vi "Actor Core.vi"(8 "error in":errorcluster, 11 "Orphan Detector in":refnum<class "Orphan Detector.lvclass">) -> (0 "error out":errorcluster, 3 "Actor out":refnum<class "Actor.lvclass">)   [LabVIEW 2017, in "MGI-Monitored Actor.lvlib" / "Orphan Detector.lvclass"]
doc: "(<B>Filename</B>: Actor Framework.lvlib:Actor.lvclass:Actor Core.vi)\n\nReceives messages to the actor, reacts to them, and initiates any error handling that may shut the actor down.\n\nDescendant classes may override this VI to append parallel tasks for the actor to complete while it handles messages. Overrides use the Call Parent Method node."
uses:
  Orphan Detector.lvclass
  <vilib>/ActorFramework/Actor/Actor.lvclass
  monitored-actor-core/Source/Monitor Data/Actor Data.ctl
  <vilib>/ActorFramework/Message Enqueuer/Message Enqueuer.lvclass
  Orphan Detector.lvclass/Orphan Detector.ctl
  <vilib>/Utility/miscctls.llb/LVRowAndColumnTypeDef.ctl
  <vilib>/ActorFramework/Message/Message.lvclass
  <vilib>/ActorFramework/Message Enqueuer/Message Enqueuer.lvclass/Message Enqueuer.ctl
  <vilib>/ActorFramework/Message Priority Queue/Priority Enqueue.vi
  monitored-actor-core/Source/Monitor Data/Monitor Data.lvclass
panel:
  in  "Poll Rate":i32=500 caption="ms"
  in  "Orphans":i32(listbox)
  # "Orphans"
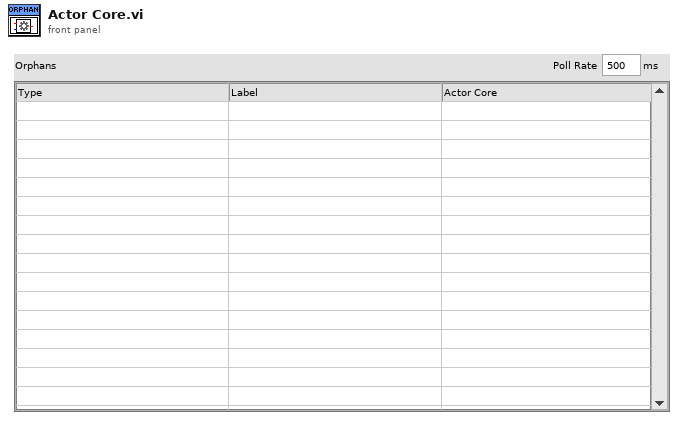
[diagram p1: front panel]
types:
  T1 = enum32{"Invalid", "Standard", "Closed", "Hidden", "Minimized", "Maximized"}
  T2 = typedef "MGI-Monitored Actor Core.lvlib/Monitor Data.lvclass/Actor Data.ctl" = cluster{"Actor Type":string, "Actor Cores":string[], "Self":refnum<class "Message Enqueuer.lvclass">, "Caller":refnum<class "Message Enqueuer.lvclass">, "Actor Label":string, "Last Ping":dbl}
  T3 = typedef "LVRowAndColumnTypeDef.ctl" = cluster{"Row":i32, "Column":i32}
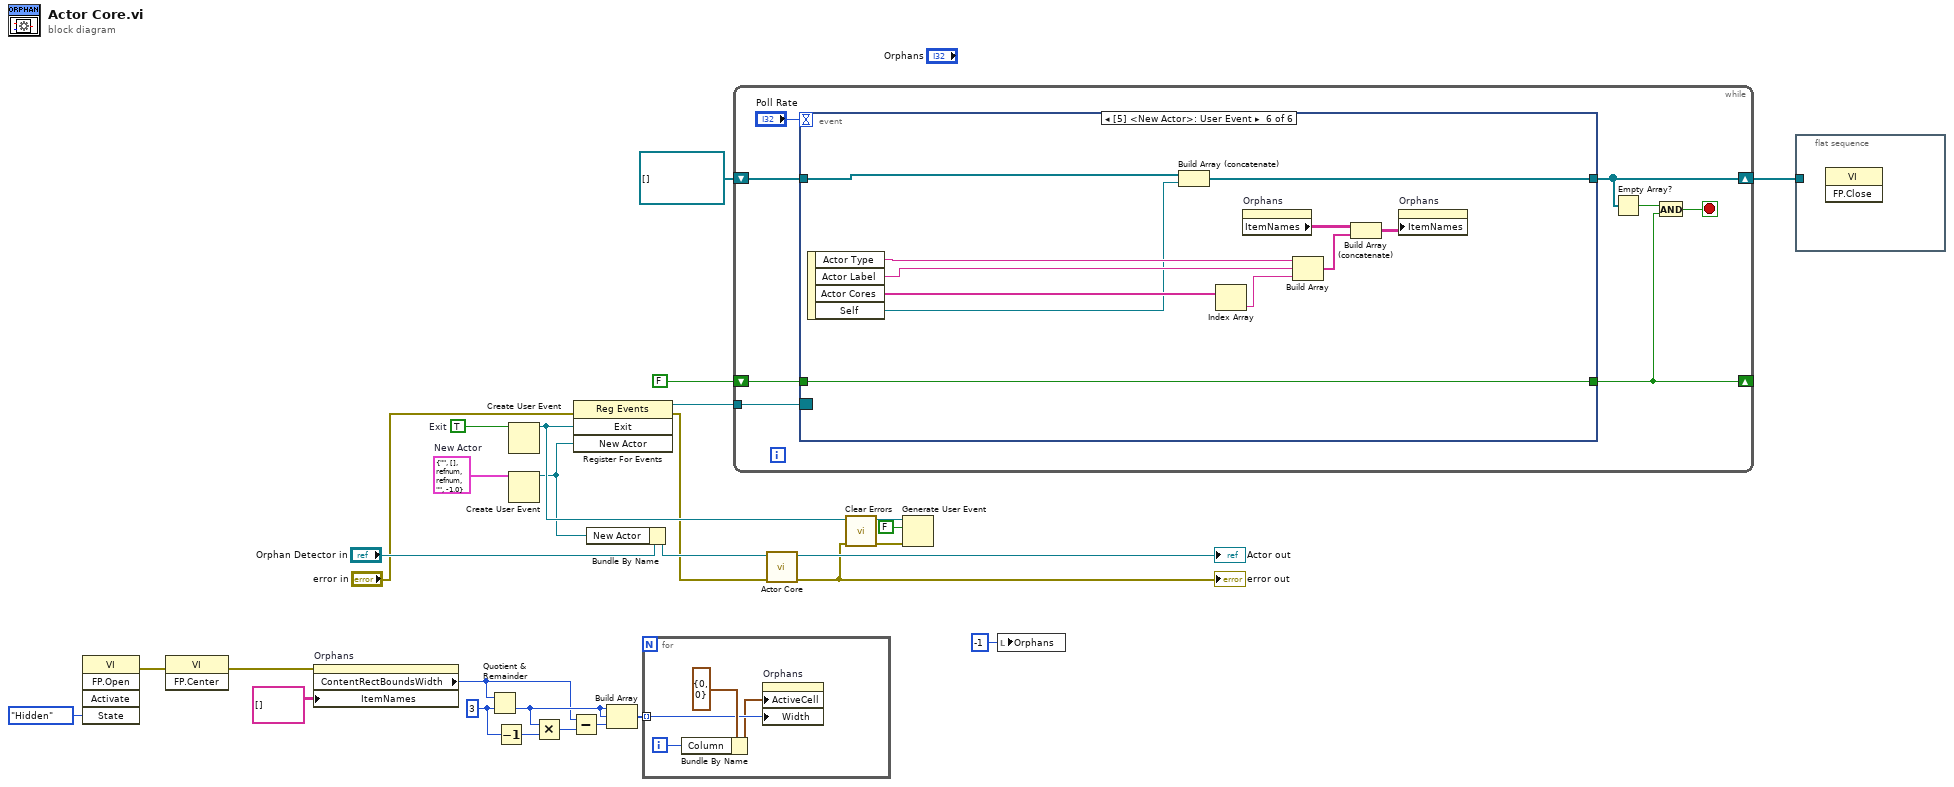
[diagram p0: block diagram]
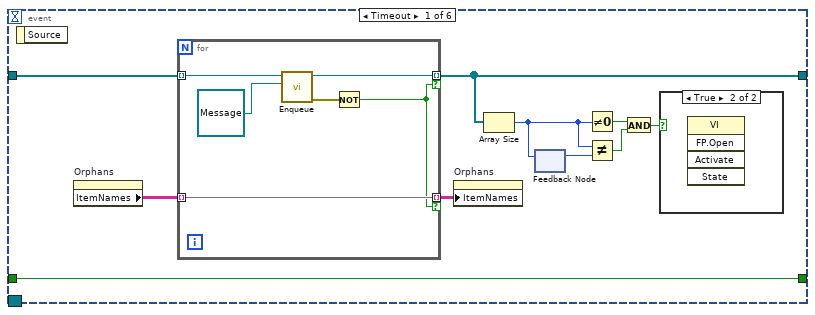
[diagram p2: hidden frame]
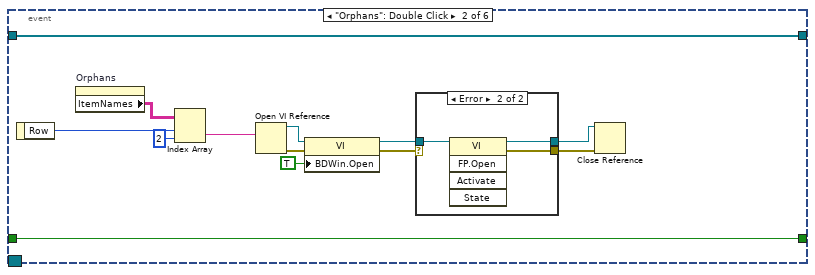
[diagram p4: hidden frame]
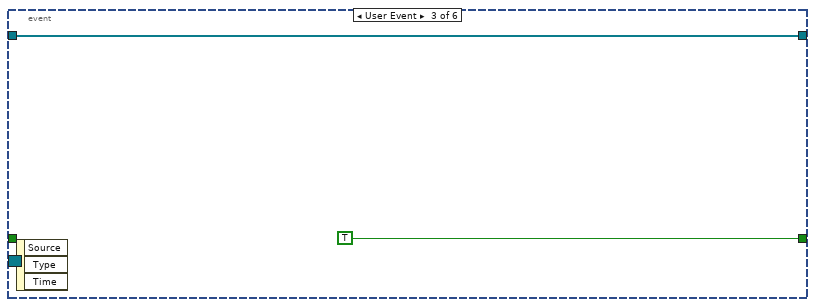
[diagram p6: hidden frame]
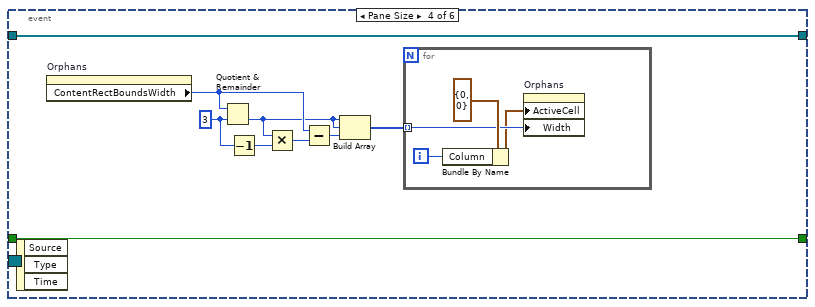
[diagram p7: hidden frame]
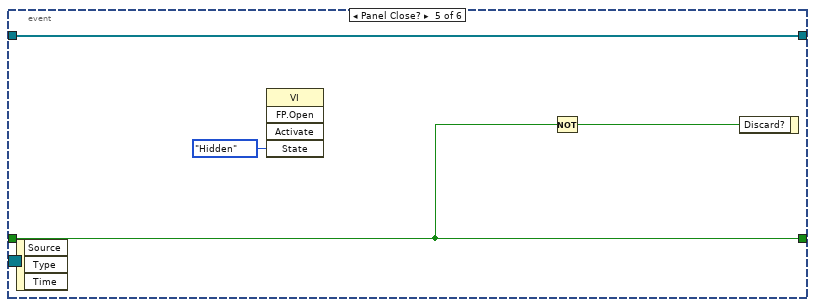
[diagram p8: hidden frame]
diagram:
  w19 = TRUE  # Exit
  w13 = T2 {"Actor Type"="", "Actor Cores"=[], "Self"=refnum, "Caller"=refnum, "Actor Label"="", "Last Ping"=-1.0}  # New Actor
  w25 = 3 ("y")
  n1 = invoke class="VI" method="FP.Open"("State"=T1."Hidden") -> (error out=w7:errorcluster)  [unwired: 4 in, 4 out]
  n2 = invoke class="VI" method="FP.Center"(error in=w7) -> (error out=w6:errorcluster)  [unwired: 2 in, 2 out]
  n3 = property on="Orphans" class="MCListbox (strict)"(error in=w6, "ItemNames"=string[][] [] ("Item Names")) -> ("ContentRectBoundsWidth"=w20:i32)  [unwired: 1 in, 2 out]
  n4 = Quotient & Remainder(x=w20, y=w25) -> (floor(x/y)=w21:i32)  [unwired: 1 out]
  n5 = Decrement(x=w25) -> (x-1=w24:i32)
  n6 = Create User Event(user event datatype=w19) -> (user event=w15:refnum<user-event>)  [unwired: 1 in, 1 out]
  n7 = Create User Event(user event datatype=w13) -> (user event=w11:refnum<user-event>)  [unwired: 1 in, 1 out]
  n8 = Multiply(x=w21, y=w24) -> (x*y=w22:i32)
  n9 = Subtract(x=w20, y=w22) -> (x-y=w26:i32)
  n10 = register-events(error in="error in", w15, w11) -> (reference out=w18:refnum<event-registration>, error out=w1:errorcluster)  [unwired: 1 in]
  n11 = Bundle By Name(cluster="Orphan Detector in", "New Actor"=w11) -> (w12:refnum<class "Orphan Detector.lvclass">)
  n12 = Build Array(w21, w21, w26) -> (w23:i32[])
  n13 = for {
    tunnel: w23 -> [w31] mode=indexing
    i -> [w29]
    n14 = Bundle By Name(cluster=T3 {"Row"=0, "Column"=0} ("Active Cell:Active Cell"), "Column"=w29) -> (w30:T3)
    n15 = property on="Orphans" class="MCListbox (strict)"("ActiveCell"=w30, "Width"=w31) -> ()  [unwired: 2 in, 2 out]
  }
  n16 = while {
    tunnel: w18 -> [w40]
    shift-right: [w36] -> w4
    shift-left: refnum<class "Message Enqueuer.lvclass">[] [] -> [w38]
    shift-right: [w34] -> _
    shift-left: FALSE -> [w37]
    stop <- w33 stop-if-true
    n17 = event shown="[5] <New Actor>: User Event" {
      selector: w40 -> [_ _ _ _ _ _]
      dyn-events: _ -> [_ _ _ _ _ _]
      timeout: "Poll Rate" -> [_ _ _ _ _ _]
      tunnel: [w47 w69 w76 w78 w93 w97] -> w36
      tunnel: w38 -> [w50 w69 w76 w78 w93 w96]
      tunnel: [w41 w65 TRUE w77 w91 w95] -> w34
      tunnel: w37 -> [w41 w65 _ w77 w91 w95]
      event Timeout {
        n18 = event-data() -> ()  [unwired: 1 in, 1 out]
        n19 = property on="Orphans" class="MCListbox (strict)"() -> ("ItemNames"=w49:string[][])  [unwired: 2 in, 2 out]
        n20 = for {
          tunnel: w50 -> [w56] mode=indexing
          tunnel: w49 -> [w53] mode=indexing
          tunnel: [w54] -> w47 mode=indexing if=w51
          tunnel: [w53] -> w48 mode=indexing if=w51
          n21 = call <vilib>:"Enqueue.vi"("Message"=refnum<class "Message.lvclass"> refnum, "Message Enqueuer in"=w56) -> ("error out"=w52:errorcluster, "Message Enqueuer out"=w54:refnum<class "Message Enqueuer.lvclass">)  [unwired: 8 in]
          n22 = Not(x=w52) -> (.not. x?=w51:bool)
        }
        n23 = property on="Orphans" class="MCListbox (strict)"("ItemNames"=w48) -> ()  [unwired: 2 in, 2 out]
        n24 = Array Size(array=w47) -> (size(s)=w45:i32)
        n25 = feedback-in #1(w45) -> ()
        n26 = feedback #1() -> (w46:i32)  [unwired: 1 in]
        n27 = Not Equal To 0?(x=w45) -> (x != 0?=w44:bool)
        n28 = Not Equal?(x=w45, y=w46) -> (x != y?=w43:bool)
        n29 = And(x=w44, y=w43) -> (x .and. y?=w42:bool)
        n30 = case shown="True" w42 {
          frame False {
          }
          frame True {
            n31 = invoke class="VI" method="FP.Open"() -> ()  [unwired: 5 in, 5 out]
          }
        }
      }
      event "Orphans": Double Click {
        n32 = event-data() -> ("Row"=w67:i32)  [unwired: 1 in]
        n33 = property on="Orphans" class="MCListbox (strict)"() -> ("ItemNames"=w68:string[][])  [unwired: 2 in, 2 out]
        n34 = Index Array(array=w68, index (row)=w67, index (col)=2 ("disabled index (col)")) -> (element=w57:string)
        n35 = Open VI Reference(vi path=w57) -> (vi reference=w64:refnum<vi>, error out=w63:errorcluster)  [unwired: 5 in]
        n36 = property class="VI"(reference=w64, error in=w63, "BDWin.Open"=TRUE ("Block Diagram Window:Open")) -> (reference out=w62:refnum<vi>, error out=w61:errorcluster)
        n37 = case shown="Error" w61 {
          selector: w61 -> [w71 _]
          tunnel: w62 -> [w70 w74]
          tunnel: [w70 w73] -> w58
          tunnel: [w71 w72] -> w59
          frame No Error {
          }
          frame Error {
            n38 = invoke class="VI" method="FP.Open"(reference=w74) -> (reference out=w73:refnum<vi>, error out=w72:errorcluster)  [unwired: 4 in, 3 out]
          }
        }
        n39 = Close Reference(reference=w58, error in (no error)=w59) -> ()  [unwired: 1 out]
      }
      event User Event {
        n40 = event-data() -> ()  [unwired: 1 in, 3 out]
      }
      event Pane Size {
        w80 = 3 ("y")
        n41 = event-data() -> ()  [unwired: 1 in, 3 out]
        n42 = property on="Orphans" class="MCListbox (strict)"() -> ("ContentRectBoundsWidth"=w85:i32)  [unwired: 2 in, 2 out]
        n43 = Quotient & Remainder(x=w85, y=w80) -> (floor(x/y)=w84:i32)  [unwired: 1 out]
        n44 = Decrement(x=w80) -> (x-1=w81:i32)
        n45 = Multiply(x=w84, y=w81) -> (x*y=w83:i32)
        n46 = Subtract(x=w85, y=w83) -> (x-y=w79:i32)
        n47 = Build Array(w84, w84, w79) -> (w82:i32[])
        n48 = for {
          tunnel: w82 -> [w88] mode=indexing
          i -> [w86]
          n49 = Bundle By Name(cluster=T3 {"Row"=0, "Column"=0} ("Active Cell:Active Cell"), "Column"=w86) -> (w87:T3)
          n50 = property on="Orphans" class="MCListbox (strict)"("ActiveCell"=w87, "Width"=w88) -> ()  [unwired: 2 in, 2 out]
        }
      }
      event Panel Close? {
        n51 = event-data() -> ()  [unwired: 1 in, 3 out]
        n52 = invoke class="VI" method="FP.Open"("State"=T1."Hidden") -> ()  [unwired: 4 in, 5 out]
        n53 = Not(x=w91) -> (.not. x?=w90:bool)
        n54 = event-data("Discard?"=w90) -> ()  [unwired: 1 in, 1 out]
      }
      event User Event {
        n55 = event-data() -> ("Actor Type"=w104:string, "Actor Label"=w103:string, "Actor Cores"=w102:string[], "Self"=w98:refnum<class "Message Enqueuer.lvclass">)  [unwired: 1 in]
        n56 = Build Array (concatenate)(w96, w98) -> (w97:refnum<class "Message Enqueuer.lvclass">[])
        n57 = Index Array(array=w102) -> (element=w94:string)  [unwired: 1 in]
        n58 = property on="Orphans" class="MCListbox (strict)"() -> ("ItemNames"=w101:string[][])  [unwired: 2 in, 2 out]
        n59 = Build Array(w104, w103, w94) -> (w99:string[])
        n60 = Build Array (concatenate)(w101, w99) -> (w100:string[][])
        n61 = property on="Orphans" class="MCListbox (strict)"("ItemNames"=w100) -> ()  [unwired: 2 in, 2 out]
      }
    }
    n62 = Empty Array?(array=w36) -> (empty?=w35:bool)
    n63 = And(x=w35, y=w34) -> (x .and. y?=w33:bool)
  }
  n64 = call-parent "Actor Core.vi"("error in"=w1, "Actor in"=w12) -> ("error out"=w17:errorcluster, "Actor out"=→"Actor out":refnum<class "Actor.lvclass">)  [unwired: 8 in]
  "error out" <- w17
  n65 = call <vilib>:"Clear Errors.vi"("error in (no error)"=w17) -> ("error out"=w16:errorcluster)  [unwired: 5 in, 1 out]
  n66 = Generate User Event(user event=w15, event data cluster=FALSE ("event data"), error in=w16) -> ()  [unwired: 1 in, 2 out]
  n67 = local write "Orphans"(-1 ("Orphans")) -> ()
  n68 = flat-sequence {
    tunnel: w4 -> [_]
    frame #0 {
      n69 = invoke class="VI" method="FP.Close"() -> ()  [unwired: 3 in, 3 out]
    }
  }
